vi "BioGas.vi"() -> ()   [LabVIEW 2019]
panel:
  out "CMD Error":string
  out "CMD Output":string
  in  "CMD Output":bool
  in  "Help Button":bool
  out "Output Files Path":path caption="selected path"
  in  "Open Button":bool
  out "# Lines Plot":i32
  out "Output File Loaded?":bool
  out "Spec File Loaded":bool
  in  "Save Specs":bool
  out "Vali File Loaded":bool
  in  "Load Spec File":bool
  in  "Load Vali File":bool
  in  "LUA Specification File":path
  in  "LUA Validation File":path
  in  "Validate":bool
  in  "Clear Plot Selection":bool
  in  "Plot":bool
  out "# Lines":i32
  in  "Parameters to Plot":string(tree)="_3"
  in  "Refresh Button":bool
  in  "Parameters":string(tree)="_3"
  in  "Run":bool
  in  "Stop":bool
  # "Biogas Control Panel"
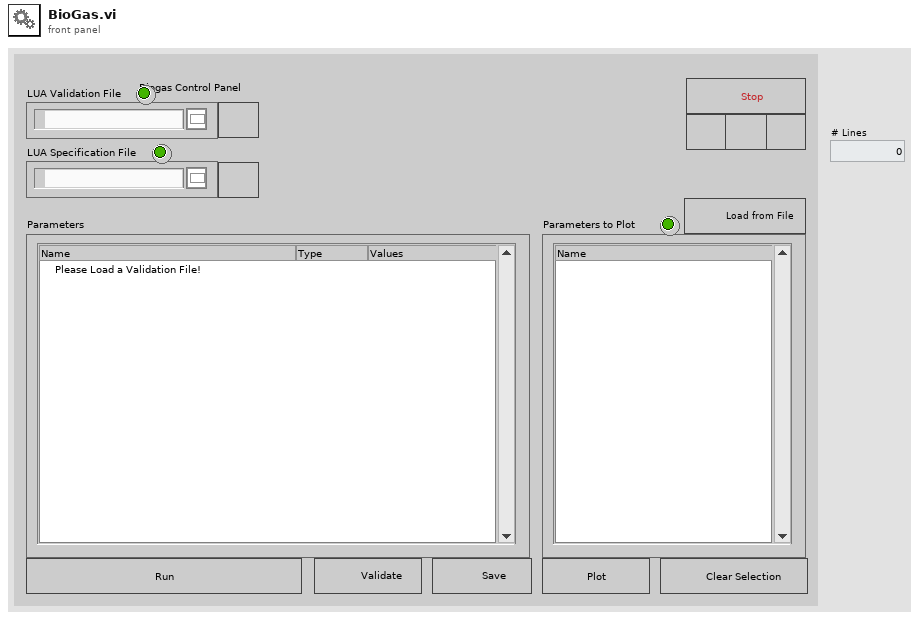
[diagram p1: front panel]
types:
  T1 = typedef "LVPoint32TypeDef.ctl" = cluster{"Horizontal":i32, "Vertical":i32}
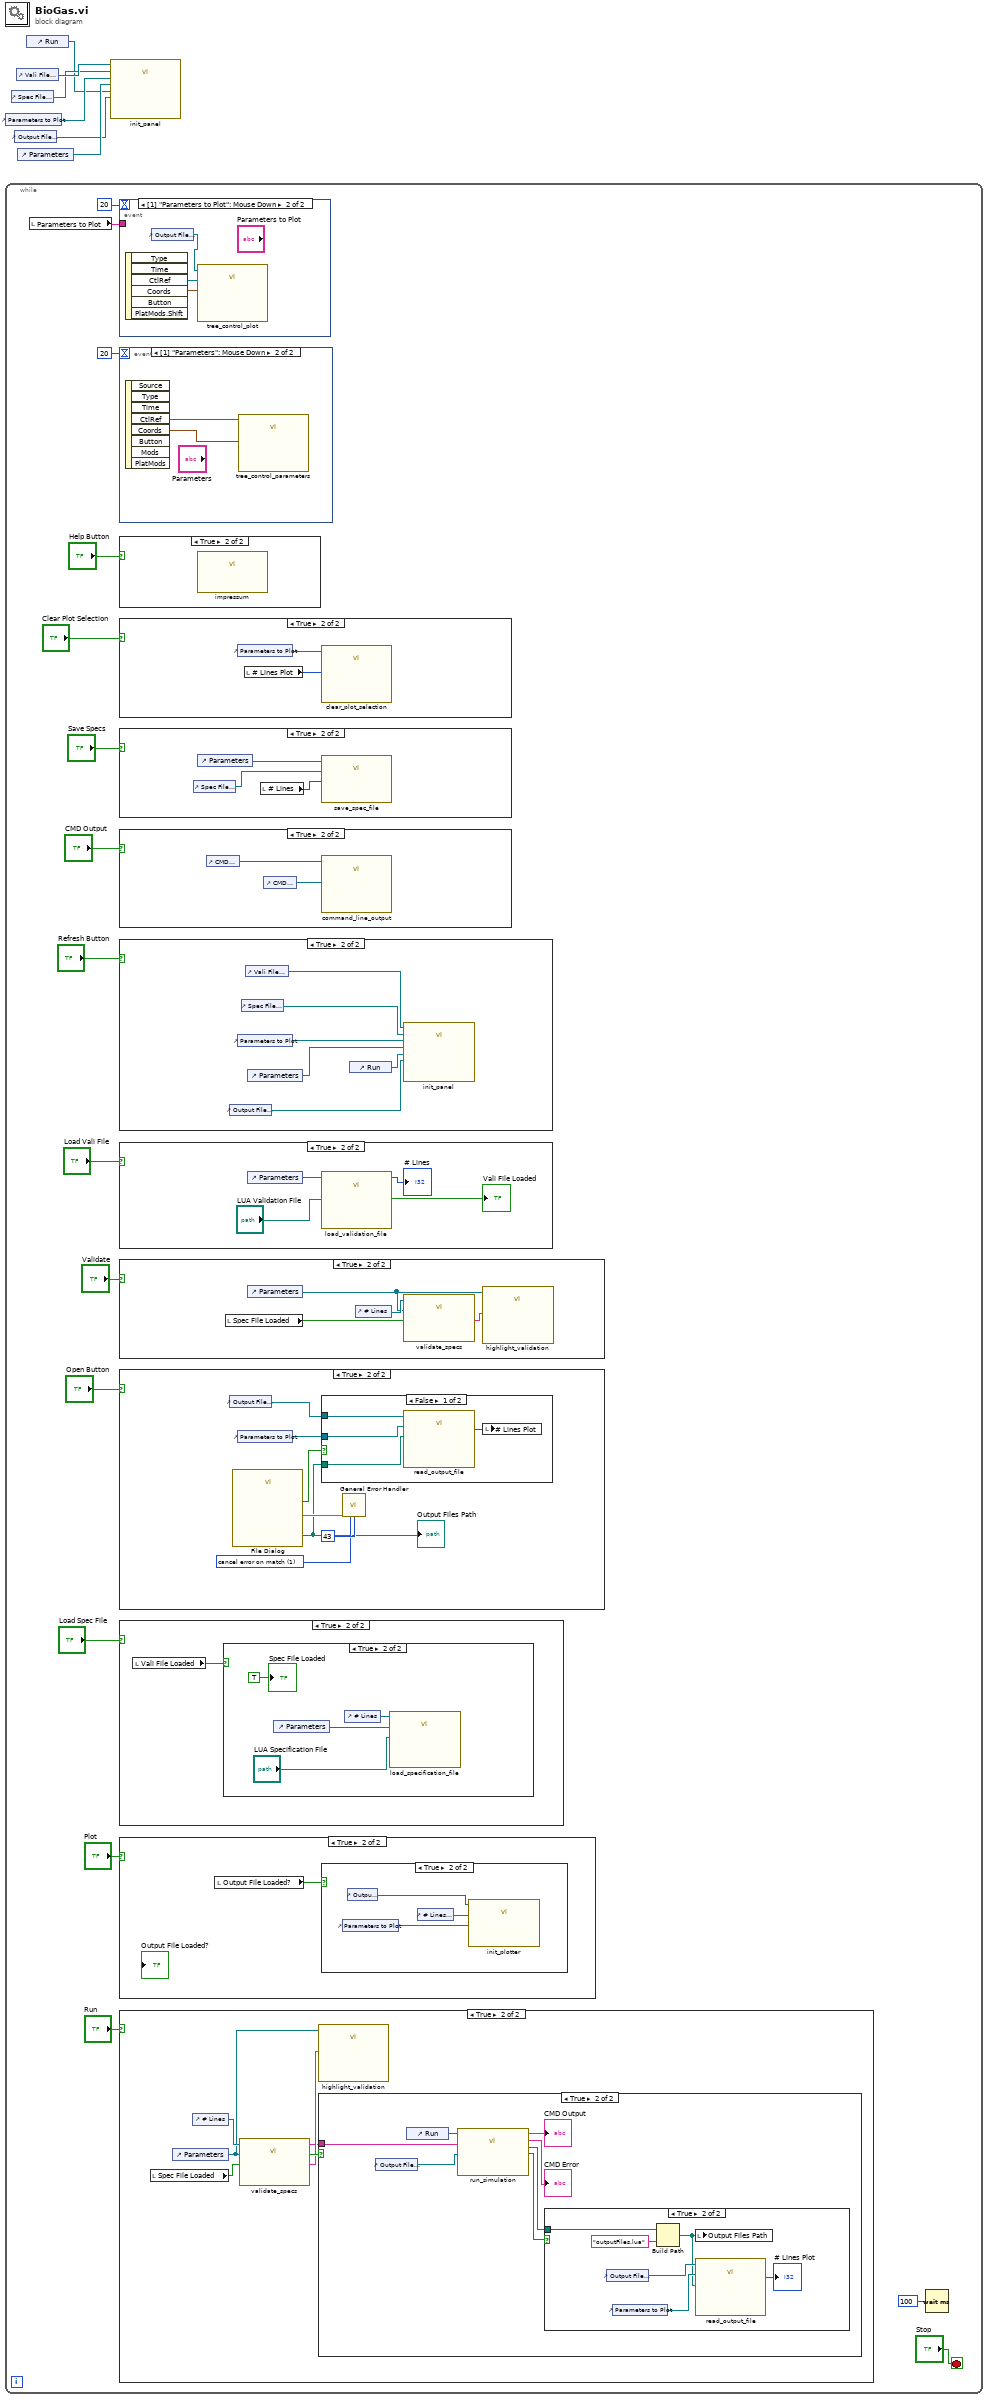
[diagram p0: block diagram]
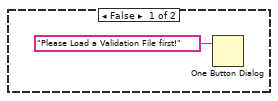
[diagram p9: hidden frame]
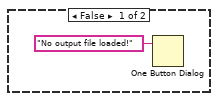
[diagram p12: hidden frame]
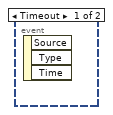
[diagram p13: hidden frame]
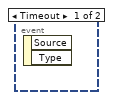
[diagram p15: hidden frame]
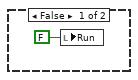
[diagram p18: hidden frame]
diagram:
  n1 = control-ref of="Parameters to Plot"() -> (w4:refnum<vi>)
  n2 = while {
    stop <- "Stop" stop-if-true
    n3 = local read "Parameters to Plot"() -> (w18:string)
    n4 = event shown="[1] \"Parameters to Plot\": Mouse Down" {
      selector: _ -> [_ _]
      dyn-events: _ -> [_ _]
      timeout: 20 -> [_ _]
      tunnel: w18 -> [_ _]
      event Timeout {
        n5 = event-data() -> ()  [unwired: 1 in, 2 out]
      }
      event "Parameters to Plot": Mouse Down {
        n6 = event-data() -> ("CtlRef"=w64:refnum<vi>, "Coords"=w63:T1)  [unwired: 1 in, 4 out]
        n7 = control-ref of="Output File Loaded?"() -> (w62:refnum<vi>)
        n8 = call "tree_control_plot.vi"("Point"=w63, "Plot Tree"=w64, "Output File Loaded?"=w62) -> ()  [unwired: 9 in]
      }
    }
    n9 = event shown="[1] \"Parameters\": Mouse Down" {
      selector: _ -> [_ _]
      dyn-events: _ -> [_ _]
      timeout: 20 -> [_ _]
      event Timeout {
        n10 = event-data() -> ()  [unwired: 1 in, 3 out]
      }
      event "Parameters": Mouse Down {
        n11 = event-data() -> ("CtlRef"=w59:refnum<vi>, "Coords"=w58:T1)  [unwired: 1 in, 6 out]
        n12 = call "tree_control_parameters.vi"("Point"=w58, "Parameters Tree"=w59) -> ()  [unwired: 10 in]
      }
    }
    n13 = case shown="True" "Help Button" {
      frame False {
      }
      frame True {
        n14 = call "impressum.vi"() -> ()  [unwired: 12 in]
      }
    }
    n15 = case shown="True" "Clear Plot Selection" {
      frame False {
      }
      frame True {
        n16 = control-ref of="Parameters to Plot"() -> (w60:refnum<vi>)
        n17 = local read "# Lines Plot"() -> (w61:i32)
        n18 = call "clear_plot_selection.vi"("# Lines Plot"=w61, "Plot Tree"=w60) -> ()  [unwired: 10 in]
      }
    }
    n19 = case shown="True" "Save Specs" {
      frame False {
      }
      frame True {
        n20 = control-ref of="Spec File Loaded"() -> (w36:refnum<vi>)
        n21 = control-ref of="Parameters"() -> (w37:refnum<vi>)
        n22 = local read "# Lines"() -> (w38:i32)
        n23 = call "save_spec_file.vi"("# Lines"=w38, "Spec File Loaded?"=w36, "Parameters Tree"=w37) -> ()  [unwired: 9 in]
      }
    }
    n24 = case shown="True" "CMD Output" {
      frame False {
      }
      frame True {
        n25 = control-ref of="CMD Output"() -> (w23:refnum<vi>)
        n26 = control-ref of="CMD Error"() -> (w24:refnum<vi>)
        n27 = call "command_line_output.vi"("CMD Error"=w24, "CMD Output"=w23) -> ()  [unwired: 10 in]
      }
    }
    n28 = case shown="True" "Refresh Button" {
      frame False {
      }
      frame True {
        n29 = control-ref of="Output File Loaded?"() -> (w66:refnum<vi>)
        n30 = control-ref of="Parameters to Plot"() -> (w68:refnum<vi>)
        n31 = control-ref of="Spec File Loaded"() -> (w67:refnum<vi>)
        n32 = control-ref of="Vali File Loaded"() -> (w70:refnum<vi>)
        n33 = control-ref of="Parameters"() -> (w69:refnum<vi>)
        n34 = control-ref of="Run"() -> (w65:refnum<vi>)
        n35 = call "init_panel.vi"("Run"=w65, "Succesfull Run"=w66, "Parameters Tree"=w69, "Plot Tree"=w68, "Spec File Loaded?"=w67, "Vali File Loaded?"=w70) -> ()  [unwired: 6 in]
      }
    }
    n36 = case shown="True" "Load Vali File" {
      frame False {
      }
      frame True {
        n37 = control-ref of="Parameters"() -> (w51:refnum<vi>)
        n38 = call "load_validation_file.vi"("LUA Validation File"="LUA Validation File", "Parameters Tree"=w51) -> ("Vali File Loaded"=→"Vali File Loaded":bool, "# Lines"=→"# Lines":i32)  [unwired: 8 in]
      }
    }
    n39 = case shown="True" "Validate" {
      frame False {
      }
      frame True {
        n40 = local read "Spec File Loaded"() -> (w42:bool)
        n41 = control-ref of="Parameters"() -> (w39:refnum<vi>)
        n42 = control-ref of="# Lines"() -> (w41:refnum<vi>)
        n43 = call "validate_specs.vi"("Spec File Loaded"=w42, "Parameters Tree"=w39, "# Lines"=w41) -> ("validationErrors"=w40:string)  [unwired: 6 in, 2 out]
        n44 = call "highlight_validation.vi"("validationErrors"=w40, "Parameters Tree"=w39) -> ()  [unwired: 10 in]
      }
    }
    n45 = case shown="True" "Open Button" {
      frame False {
      }
      frame True {
        w29 = 1 items=["no exception", "cancel error on match", "set error on match"] ("[exception action] (none:0)")
        n46 = control-ref of="Output File Loaded?"() -> (w25:refnum<vi>)
        n47 = call "File Dialog"() -> ("selected path"=w27:path, "cancelled"=w28:bool, "error out"=w31:errorcluster)  [unwired: 12 in, 1 out]
        "Output Files Path" <- w27
        n48 = control-ref of="Parameters to Plot"() -> (w26:refnum<vi>)
        n49 = case shown="False" w28 {
          tunnel: w27 -> [w35 _]
          tunnel: w26 -> [w34 _]
          tunnel: w25 -> [w32 _]
          frame False {
            n50 = call "read_output_file.vi"("TMP Filepath"=w35, "Plot Tree"=w34, "Output File Loaded?"=w32) -> ("# Lines Plot"=w33:i32)  [unwired: 8 in]
            n51 = local write "# Lines Plot"(w33) -> ()
          }
          frame True {
          }
        }
        n52 = call <vilib>:"General Error Handler.vi"("error in (no error)"=w31, "[exception action] (none:0)"=w29, "[exception code]"=43) -> ()  [unwired: 8 in, 5 out]
      }
    }
    n53 = case shown="True" "Load Spec File" {
      frame False {
      }
      frame True {
        n54 = local read "Vali File Loaded"() -> (w43:bool)
        n55 = case shown="True" w43 {
          frame False {
            n56 = One Button Dialog(message="Please Load a Validation File first!") -> ()  [unwired: 1 in, 1 out]
          }
          frame True {
            n57 = control-ref of="Parameters"() -> (w46:refnum<vi>)
            n58 = control-ref of="# Lines"() -> (w47:refnum<vi>)
            n59 = call "load_specification_file.vi"("LUA Specification File"="LUA Specification File", "Parameters Tree"=w46, "Digital in"=w47) -> ()  [unwired: 9 in]
            "Spec File Loaded" <- TRUE ("Spec File Loaded")
          }
        }
      }
    }
    n60 = case shown="True" "Plot" {
      frame False {
      }
      frame True {
        n61 = local read "Output File Loaded?"() -> (w53:bool)
        n62 = case shown="True" w53 {
          frame False {
            n63 = One Button Dialog(message="No output file loaded!") -> ()  [unwired: 1 in, 1 out]
          }
          frame True {
            n64 = control-ref of="Parameters to Plot"() -> (w55:refnum<vi>)
            n65 = control-ref of="Output Files Path"() -> (w57:refnum<vi>)
            n66 = control-ref of="# Lines Plot"() -> (w56:refnum<vi>)
            n67 = call "init_plotter.vi"("Plot Tree"=w55, "#Lines Plot"=w56, "Output Files Path"=w57) -> ()  [unwired: 9 in]
          }
        }
      }
    }
    n68 = case shown="True" "Run" {
      frame False {
      }
      frame True {
        n69 = local read "Spec File Loaded"() -> (w75:bool)
        n70 = control-ref of="Parameters"() -> (w73:refnum<vi>)
        n71 = control-ref of="# Lines"() -> (w76:refnum<vi>)
        n72 = call "validate_specs.vi"("Spec File Loaded"=w75, "Parameters Tree"=w73, "# Lines"=w76) -> ("validationErrors"=w72:string, "Valid?"=w74:bool, "Specifications"=w71:string)  [unwired: 6 in]
        n73 = call "highlight_validation.vi"("validationErrors"=w72, "Parameters Tree"=w73) -> ()  [unwired: 10 in]
        n74 = case shown="True" w74 {
          tunnel: w71 -> [_ w78]
          frame False {
            n75 = local write "Run"(FALSE ("Run")) -> ()
          }
          frame True {
            n76 = control-ref of="Output File Loaded?"() -> (w83:refnum<vi>)
            n77 = control-ref of="Run"() -> (w84:refnum<vi>)
            n78 = call "run_simulation.vi"("Output File Loaded?"=w83, "inputSpecs"=w78, "Run"=w84) -> ("OK"=w82:bool, "TMP Filepath"=w81:path, "standard error"=→"CMD Error":string, "standard output"=→"CMD Output":string)  [unwired: 5 in]
            n79 = case shown="True" w82 {
              tunnel: w81 -> [_ w89]
              frame False {
              }
              frame True {
                n80 = control-ref of="Output File Loaded?"() -> (w86:refnum<vi>)
                n81 = control-ref of="Parameters to Plot"() -> (w90:refnum<vi>)
                n82 = Build Path(base path=w89, name or relative path="outputFiles.lua") -> (appended path=w85:path)
                n83 = local write "Output Files Path"(w85) -> ()
                n84 = call "read_output_file.vi"("TMP Filepath"=w85, "Plot Tree"=w90, "Output File Loaded?"=w86) -> ("# Lines Plot"=→"# Lines Plot":i32)  [unwired: 8 in]
              }
            }
          }
        }
      }
    }
    n85 = Wait (ms)(milliseconds to wait=u32 100) -> ()  [unwired: 1 out]
  }
  n86 = control-ref of="Spec File Loaded"() -> (w3:refnum<vi>)
  n87 = control-ref of="Output File Loaded?"() -> (w2:refnum<vi>)
  n88 = control-ref of="Vali File Loaded"() -> (w6:refnum<vi>)
  n89 = control-ref of="Parameters"() -> (w5:refnum<vi>)
  n90 = control-ref of="Run"() -> (w1:refnum<vi>)
  n91 = call "init_panel.vi"("Run"=w1, "Succesfull Run"=w2, "Parameters Tree"=w5, "Plot Tree"=w4, "Spec File Loaded?"=w3, "Vali File Loaded?"=w6) -> ()  [unwired: 6 in]
